vi "VI Server_TextRing_Update_ItemNames_FromSpeadsheetString.vi"(6 "Strings []: SpreadsheetFormat":string, 7 "Label":string, 8 "error in":errorcluster, 11 "VI Server Cluster":T1) -> (0 "error out":errorcluster, 1 "Control Reference":refnum<vi>, 3 "VI Server Cluster.DUP":T1)   [LabVIEW 2020, in "VI Server Toolkit LV2013.lvlib"]
doc: "Updates Text Ring Items List from spreadsheet string (comma-delimited)."
uses:
  VI Server Toolkit LV2013.lvlib
  VI Server_TypeDefs/VI Server_RefsCluster.ctl
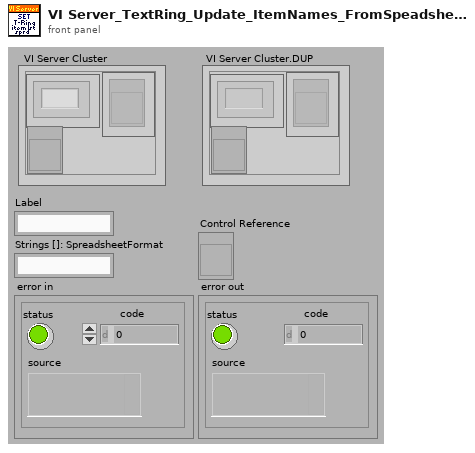
[diagram p1: front panel]
types:
  T1 = typedef "VI Server_RefsCluster.ctl" = cluster{"Labels":string[], "Refs":refnum<vi>[], "VI Ref":refnum<vi>}
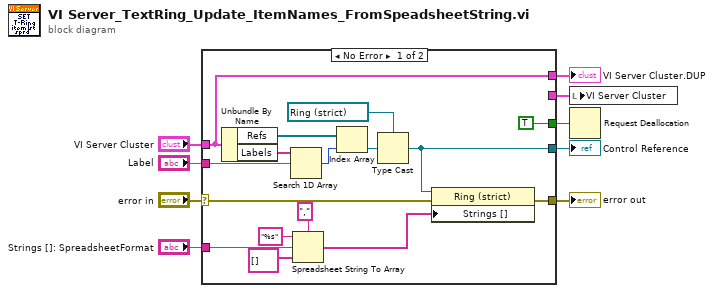
[diagram p0: block diagram]
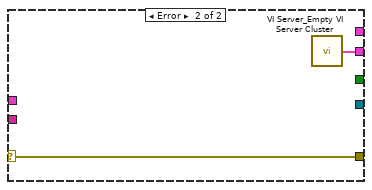
[diagram p2: hidden frame]
diagram:
  n1 = case shown="No Error" "error in" {
    selector: "error in" -> [w19 w27]
    tunnel: "Label" -> [w24 _]
    tunnel: "VI Server Cluster" -> [w11 _]
    tunnel: [w18 w27] -> w9
    tunnel: [w17 _] -> w5
    tunnel: "Strings []: SpreadsheetFormat" -> [w16 _]
    tunnel: [w11 _] -> w3
    tunnel: [TRUE _] -> w2
    tunnel: [_ w26] -> w1
    frame No Error {
      n2 = Unbundle By Name(w11) -> ("Refs"=w22:refnum<vi>[], "Labels"=w25:string[])
      n3 = Search 1D Array(1D array=w25, element=w24) -> (index of element=w23:i32)  [unwired: 1 out]
      n4 = Spreadsheet String To Array(delimiter (Tab)=",", format string="%s", spreadsheet string=w16, array type (2D Dbl)=string[] []) -> (array=w12:string[])
      n5 = Index Array(array=w22, index=w23) -> (element=w21:refnum<vi>)
      n6 = Type Cast(type=refnum<vi> refnum ("Ring"), x=w21) -> (*(type *) &x=w17:refnum<vi>)
      n7 = property class="Ring (strict)"(reference=w17, error in=w19, "Strings []"=w12) -> (error out=w18:errorcluster)  [unwired: 1 out]
    }
    frame Error {
      n8 = call "VI Server_Empty VI Server Cluster.vi"() -> ("VI Server Cluster"=w26:T1)  [unwired: 7 in]
    }
  }
  "error out" <- w9
  "VI Server Cluster.DUP" <- w3
  "Control Reference" <- w5
  n9 = local write "VI Server Cluster"(w1) -> ()
  n10 = Request Deallocation(w2) -> ()
